vi "MCP2221_Dll.vi"() -> (0 "dll path":path)   [LabVIEW 2025]
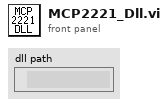
[diagram p1: front panel]
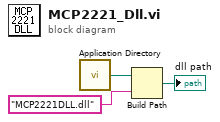
[diagram p0: block diagram]
diagram:
  n1 = call <vilib>:"Application Directory.vi"() -> ("Application Directory"=w3:path)
  n2 = Build Path(base path=w3, name or relative path="MCP2221DLL.dll") -> (appended path=→"dll path":path)
